vi "Get IO Config Path old.vi"(8 "error in (no error)":errorcluster) -> (0 "error out":errorcluster, 1 "DO COnfig path":path, 2 "DI Config path":path, 3 "AO Config path":path, 5 "AI Config path":path)   [LabVIEW 2018]
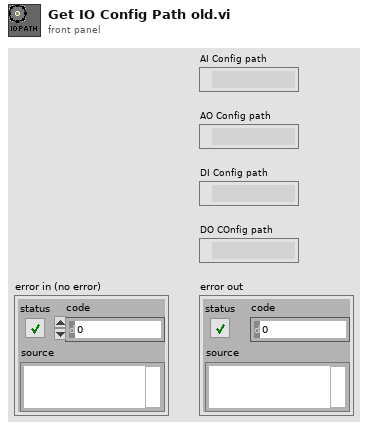
[diagram p1: front panel]
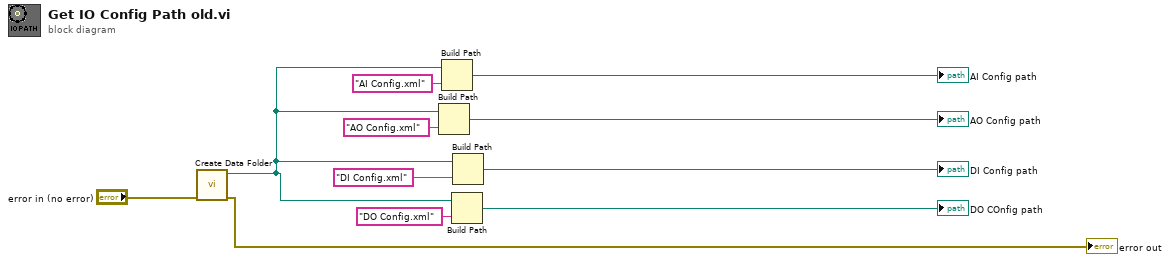
[diagram p0: block diagram]
diagram:
  n1 = call "Create Data Folder.vi"("error in (no error)"="error in (no error)") -> ("error out"=→"error out":errorcluster, "Data path"=w10:path)  [unwired: 9 in]
  n2 = Build Path(base path=w10, name or relative path="AO Config.xml") -> (appended path=→"AO Config path":path)
  n3 = Build Path(base path=w10, name or relative path="AI Config.xml") -> (appended path=→"AI Config path":path)
  n4 = Build Path(base path=w10, name or relative path="DO Config.xml") -> (appended path=→"DO COnfig path":path)
  n5 = Build Path(base path=w10, name or relative path="DI Config.xml") -> (appended path=→"DI Config path":path)
